vi "Read N Images from Buffer.vi"(8 "Error In":errorcluster, 9 "timeout (-1 = wait forever)":i32 format="%d ms", 10 "count (-1 = all)":i32=-1, 11 "reference in":refnum<class "Camera.lvclass">) -> (0 "Error Out":errorcluster, 2 "images":refnum<class "Generic Image.lvclass">[](array[class]), 3 "reference out":refnum<class "Camera.lvclass">)   [LabVIEW 2025, in "Camera.lvclass"]
uses:
  Camera.lvclass
  Typedefs/Generic Image/Generic Image.lvclass
  Camera Worker Messages/Get N Images Msg/Get N Images Msg.lvclass/Get N Images Msg.ctl
  <vilib>/ActorFramework/Specialty Messages/Reply Msg/Reply Msg.lvclass/Reply Msg.ctl
  <vilib>/ActorFramework/Message Enqueuer/Message Enqueuer.lvclass/Message Enqueuer.ctl
  <vilib>/ActorFramework/Specialty Messages/Reply Msg/Send Message And Wait For Response.vi
  <vilib>/ActorFramework/Message Enqueuer/Enqueue.vi
  Camera Worker Messages/Get N Images Msg/Get N Images Msg.lvclass
  C:/Program Files/National Instruments/LabVIEW 2025/vi.lib/ActorFramework/Specialty Messages/Reply Msg/Reply Msg.lvclass
  <vilib>/ActorFramework/Specialty Messages/Reply Msg/Reply Msg.lvclass
  C:/Program Files/National Instruments/LabVIEW 2025/vi.lib/ActorFramework/Message/Message.lvclass
  <vilib>/Utility/LVClass/Get LV Class Name.vi
  <vilib>/ActorFramework/tracing/Trace Generation/Generate Trace for Message.vi
  <vilib>/ActorFramework/Message Priority Queue/Priority Enqueue.vi
panel:
  out "timed out?":bool
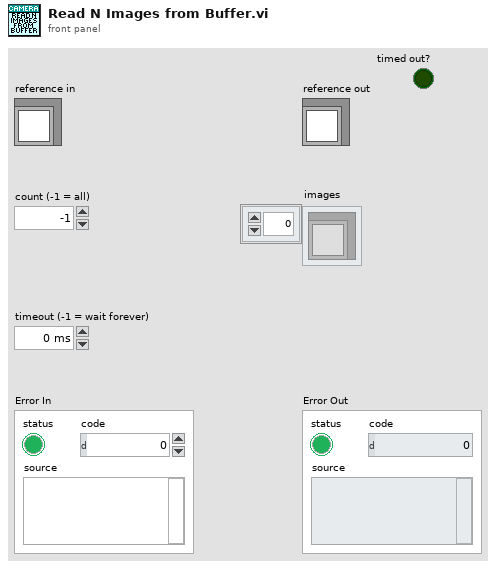
[diagram p1: front panel]
types:
  T1 = typedef "Camera.lvclass/ObjectAttributes.ctl" = cluster{"IConfigure":refnum<class "IConfigure.lvclass">, "Worker Enqueuer":refnum<class "Message Enqueuer.lvclass">, "Start Counter":i32, "Initialized":bool}
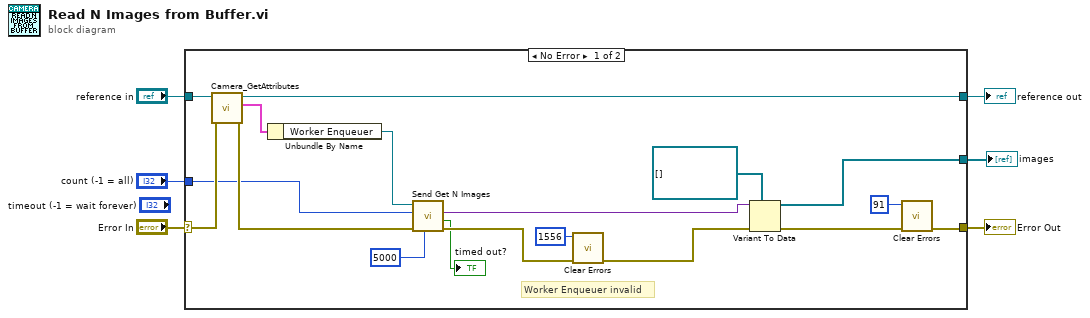
[diagram p0: block diagram]
diagram:
  n1 = case shown="No Error" "Error In" {
    selector: "Error In" -> [w24 w26]
    tunnel: [w10 w26] -> w5
    tunnel: [w22 w25] -> w3
    tunnel: "reference in" -> [w23 w25]
    tunnel: "count (-1 = all)" -> [w12 _]
    tunnel: [w15 _] -> w1
    frame No Error {
      # "Worker Enqueuer invalid"
      n2 = call "Camera_GetAttributes.vi"("Error In"=w24, "reference in"=w23) -> ("Error Out"=w18:errorcluster, "Data"=w17:T1, "reference out"=w22:refnum<class "Camera.lvclass">)  [unwired: 6 in, 1 out]
      n3 = Unbundle By Name(w17) -> ("Worker Enqueuer"=w21:refnum<class "Message Enqueuer.lvclass">)
      n4 = call "Send Get N Images.vi"("timeout in ms (-1)"=5000, "error in"=w18, "count (-1 = all)"=w12, "Message Enqueuer"=w21) -> ("error out"=w20:errorcluster, "timed out?"=→"timed out?":bool, "Reply"=w14:variant)  [unwired: 4 in, 1 out]
      n5 = call <vilib>:"Clear Errors.vi"("error in (no error)"=w20, "specific error code to clear (0: all)"=1556) -> ("error out"=w8:errorcluster)  [unwired: 4 in, 1 out]
      n6 = Variant To Data(error in=w8, type=refnum<class "Generic Image.lvclass">[] [], Variant=w14) -> (data=w15:refnum<class "Generic Image.lvclass">[], error out=w16:errorcluster)
      n7 = call <vilib>:"Clear Errors.vi"("error in (no error)"=w16, "specific error code to clear (0: all)"=91) -> ("error out"=w10:errorcluster)  [unwired: 4 in, 1 out]
    }
    frame Error {
    }
  }
  "Error Out" <- w5
  "reference out" <- w3
  "images" <- w1
